vi "Start Figure.vi"(4 "Y scale label (amplitude (V))":string="amplitude(V)", 6 "X scale label (time(s))":string="time (s)", 7 "Plot name (sampled signal)":string="sampled signal", 8 "error in (no error)":errorcluster) -> (0 "error out":errorcluster, 2 "figure reference out":refnum<vi>, 3 "queue out":refnum<queue>)   [LabVIEW 2020]
panel:
  in  "Data name (samples)":string
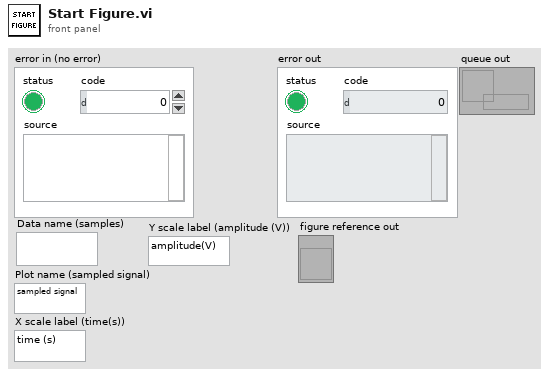
[diagram p1: front panel]
types:
  T1 = enum32{"Invalid", "Standard", "Closed", "Hidden", "Minimized", "Maximized"}
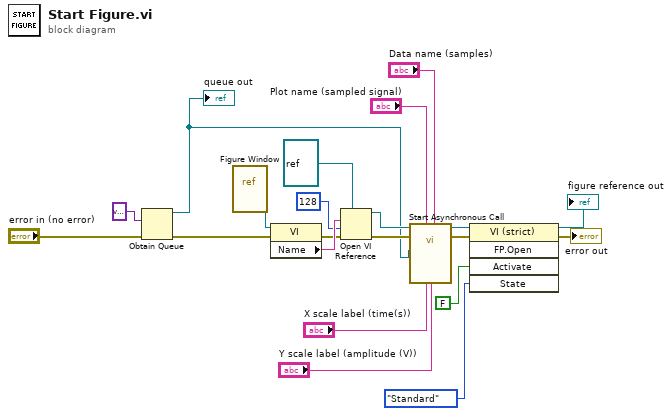
[diagram p0: block diagram]
diagram:
  n1 = Obtain Queue(element data type=variant, error in (no error)="error in (no error)") -> (queue out=w1:refnum<queue>, error out=w2:errorcluster)  [unwired: 3 in, 1 out]
  "queue out" <- w1
  n2 = vi-ref "Figure Window.vi"() -> (w20:refnum<vi>)
  n3 = property class="VI"(reference=w20, error in=w2) -> (error out=w18:errorcluster, "Name"=w19:string)  [unwired: 1 out]
  n4 = Open VI Reference(type specifier VI Refnum (for type only)=refnum<vi> refnum, vi path=w19, options=128, error in (no error)=w18) -> (vi reference=w15:refnum<vi>, error out=w14:errorcluster)  [unwired: 2 in]
  n5 = call-by-ref "Start Asynchronous Call"(reference=w15, error in=w14, "Y scale label (amplitude (V))"="Y scale label (amplitude (V))", "Data name (samples)"="Data name (samples)", "X scale label (time(s))"="X scale label (time(s))", "Plot name (sampled signal)"="Plot name (sampled signal)", "data qeue"=w1) -> (reference out=w13:refnum<vi>, error out=w12:errorcluster)  [unwired: 7 in]
  n6 = invoke class="VI (strict)" method="FP.Open"(reference=w13, error in=w12, "Activate"=FALSE ("Activate?"), "State"=T1."Standard") -> (reference out=→"figure reference out":refnum<vi>, error out=→"error out":errorcluster)  [unwired: 1 in, 3 out]
